vi "Read byte index.vi"(8 "error in":errorcluster, 11 "EthernetIP Channel in":refnum<class "EthernetIP Channel.lvclass">) -> (0 "error out":errorcluster, 2 "element number":i32, 3 "EthernetIP Channel out":refnum<class "EthernetIP Channel.lvclass">)   [LabVIEW 2013, in "EthernetIP Channel.lvclass"]
uses:
  EthernetIP Channel.lvclass
  EthernetIP Channel.lvclass/EthernetIP Channel.ctl
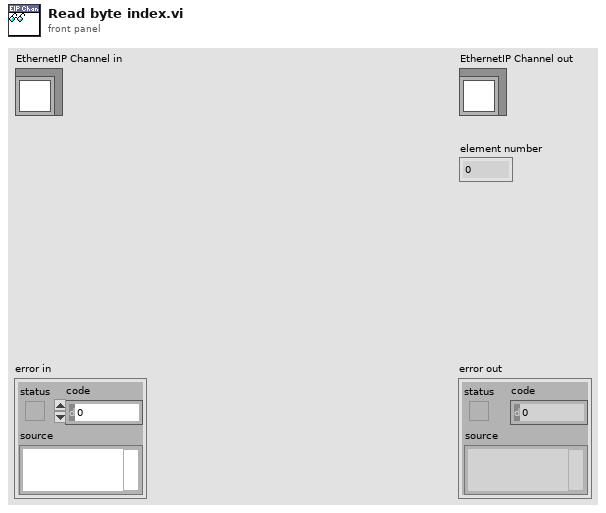
[diagram p1: front panel]
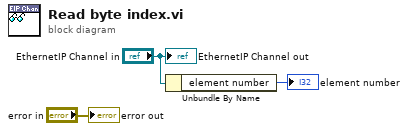
[diagram p0: block diagram]
diagram:
  n1 = Unbundle By Name("EthernetIP Channel in") -> ("element number"=→"element number":i32)
  "error out" <- "error in"
  "EthernetIP Channel out" <- "EthernetIP Channel in"
